vi "Motion-MoveXAndYNOAV.vi"(8 "error in (no error)":errorcluster, 9 "X Coordinates":string="-880000", 10 "Y Coordinates":string="880000", 11 "Motion-ControlAll in":refnum<class "Motion-ControlAll.lvclass">) -> (0 "error out":errorcluster, 3 "Motion-ControlAll out":refnum<class "Motion-ControlAll.lvclass">)   [LabVIEW 2013, in "Motion-ControlAll.lvclass"]
uses:
  Motion-ControlAll.lvclass
  Motion-ControlAll.lvclass/Motion-ControlAll.ctl
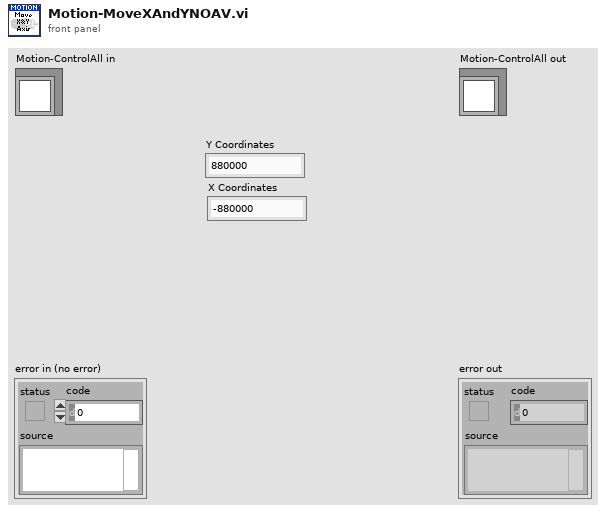
[diagram p1: front panel]
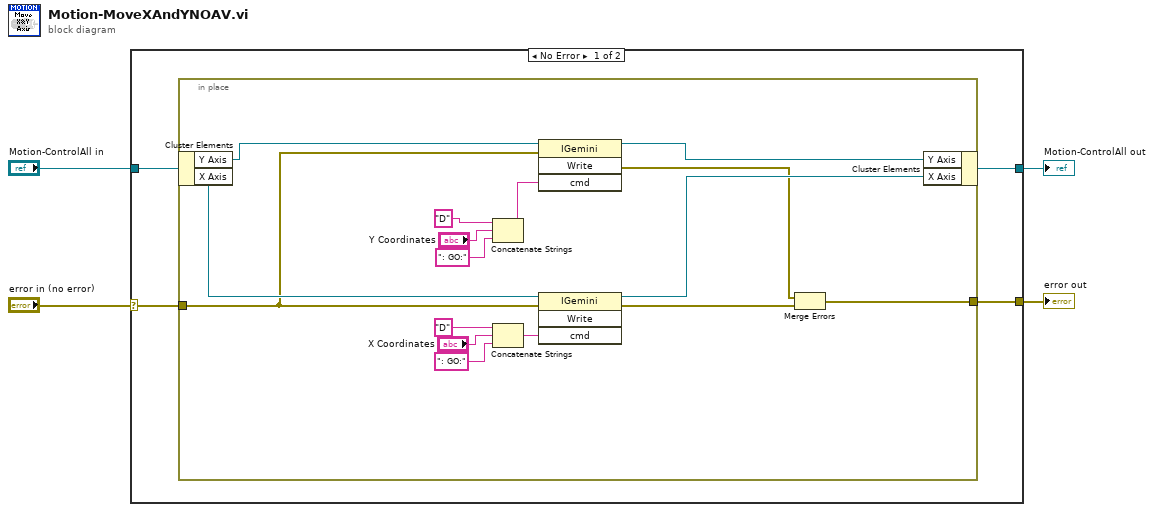
[diagram p0: block diagram]
diagram:
  n1 = case shown="No Error" "error in (no error)" {
    selector: "error in (no error)" -> [w8 w26]
    tunnel: [w7 w26] -> w3
    tunnel: [w6 w25] -> w1
    tunnel: "Motion-ControlAll in" -> [w5 w25]
    frame No Error {
      n2 = in-place {
        in-place-border: w8 -> [w17]
        in-place-border: [w11] -> w7
        n3 = in-place-cluster #1(w5) -> ("Y Axis"=w16:refnum<k7>, "X Axis"=w21:refnum<k7>)
        n4 = Concatenate Strings("D" ("string"), "Y Coordinates", ": GO:" ("string")) -> (w20:string)
        n5 = Concatenate Strings("D" ("string"), "X Coordinates", ": GO:" ("string")) -> (w22:string)
        n6 = invoke class="IGemini" method="Write"(reference=w16, error in=w17, "cmd"=w20) -> (reference out=w15:refnum<k7>, error out=w12:errorcluster)  [unwired: 1 in, 2 out]
        n7 = invoke class="IGemini" method="Write"(reference=w21, error in=w17, "cmd"=w22) -> (reference out=w14:refnum<k7>, error out=w13:errorcluster)  [unwired: 1 in, 2 out]
        n8 = Merge Errors(w12, w13) -> (w11:errorcluster)
        n9 = in-place-cluster #1("Y Axis"=w15, "X Axis"=w14) -> (w6:refnum<class "Motion-ControlAll.lvclass">)
      }
    }
    frame Error {
    }
  }
  "error out" <- w3
  "Motion-ControlAll out" <- w1
